vi "ArduPilot GCS.vi"() -> ()   [LabVIEW 8.6]
uses:
  user32.dll
  EventHandlerEnum.ctl
  Engines/SettingsEngine/SettingsEngineEnum.ctl
  EnumComm.ctl
  Engines/LogEngine/EnumLog.ctl
  Engines/SpeachEngine/EnumSpeak.ctl
panel:
  out "IMU":bool
  out "Climb Rate":dbl(knob) scale=-10.0..10.0 scale format="%#.2g"
  out "Mode":string
  out "WP":i32
  out "DistanceWP":i32 format="%.0f m"
  out "UAV Longitude":dbl format="%.6g°"
  out "UAV Latitude":dbl format="%.6g°"
  out "Throttle":i32(slide) scale=0.0..125.0
  out "Battery":dbl(slide) scale=0.0..10.0
  out "error outint comp manually":errorcluster
  out "error out clen-up":errorcluster
  out "Roll-old":i32
  out "Pitch-old":i32
  in  "WebBrowser 2":refnum<k7>(container)
  in  "Heading":string="0"
  in  "Range":string="1000"
  in  "Tilt":string="0"
  in  "Send":bool
  in  "write buffer":string
  in  "Baud Rate":string(combo)="9600"
  in  "COM Port":refnum<visa-resource-name>
  out "Comm Status":bool
  in  "EARTHLib.IApplicationGE":refnum<k7>
  in  "EARTHLib.IKHInterface":refnum<k7>
  out "GPS fix":bool
  out "error out":errorcluster
  out "StatusMsg":string
  out "Ground Speed Num":i32 format="%.0f m/s"
  out "Air Speed Num":i32 format="%.0f m/s"
  in  "Stop":bool
  out "Est Time Left":i32
  out "Amps":i32
  out "Watts":i32
  out "log data":string
  in  "Tab Control":T1(tab)
  out "GndSpeed":i32(knob) scale=0.0..50.0
  out "AS":i32
  out "GS":i32
  out "AirSpeed":i32(knob) caption="Air Speed" scale=0.0..50.0
  out "Roll Ind":cluster{i32, i32}(knob)={0, 180} scale=0.0..360.0
  out "Pitch-pic":picture
  out "Course   Bearing":cluster{i32, i32}(knob) scale=0.0..360.0 scale format="%.0f°"
  out "Altitude":cluster{i32, i32}(knob) scale=0.0..200.0
  out "BER":i32
  out "CRS":i32
  out "ALT":i32
  out "ALH":i32
  out "Roll":i32
  out "Pitch":i32
  in  "Zoom":u16(slide)=1000 scale=60000.0..1.0
  in  "Tilt":u8(slide) scale=0.0..90.0
  in  "Connect":bool
  in  "Baud Rate -M":string(combo)="9600"
  in  "COM Port -M":refnum<visa-resource-name>
  in  "kml write interval [s]":u32=1
  in  "Announcement interval [sec]":u32=30
  in  "Pan":i16(knob) scale=0.0..359.0
  out "IMU Performance data":string
  out "IMU health":i32
  out "Debug / Not Telemetry Data":string
  out "Raw Data":string
  # "NOT USED"
  # "%%%PWP:\t\t376322464,\t-1224913280,\t300,\nNWP:0,\t376321530,\t-1224913400,\t1200,***"
  # "meters"
  # "Climb Rate"
  # "lon 122\nlat 37"
  # "-122.491"
  # "37.6322"
  # "meters"
  # "ALH"
  # "m / s"
  # "meters"
  # "ALH"
  # "Gnd Speed"
  # "m/s"
  # "AP port - manuall connection"
  # "To manually connect to AP serial port\nselect desired 'COM port' and 'Boud Rate' values\nand press 'Connect'"
  # "Google Earth Controls"
  # "Audio"
  # "N"
  # "(How often to update kml (GE) display)"
  # "Received"
  # "Set"
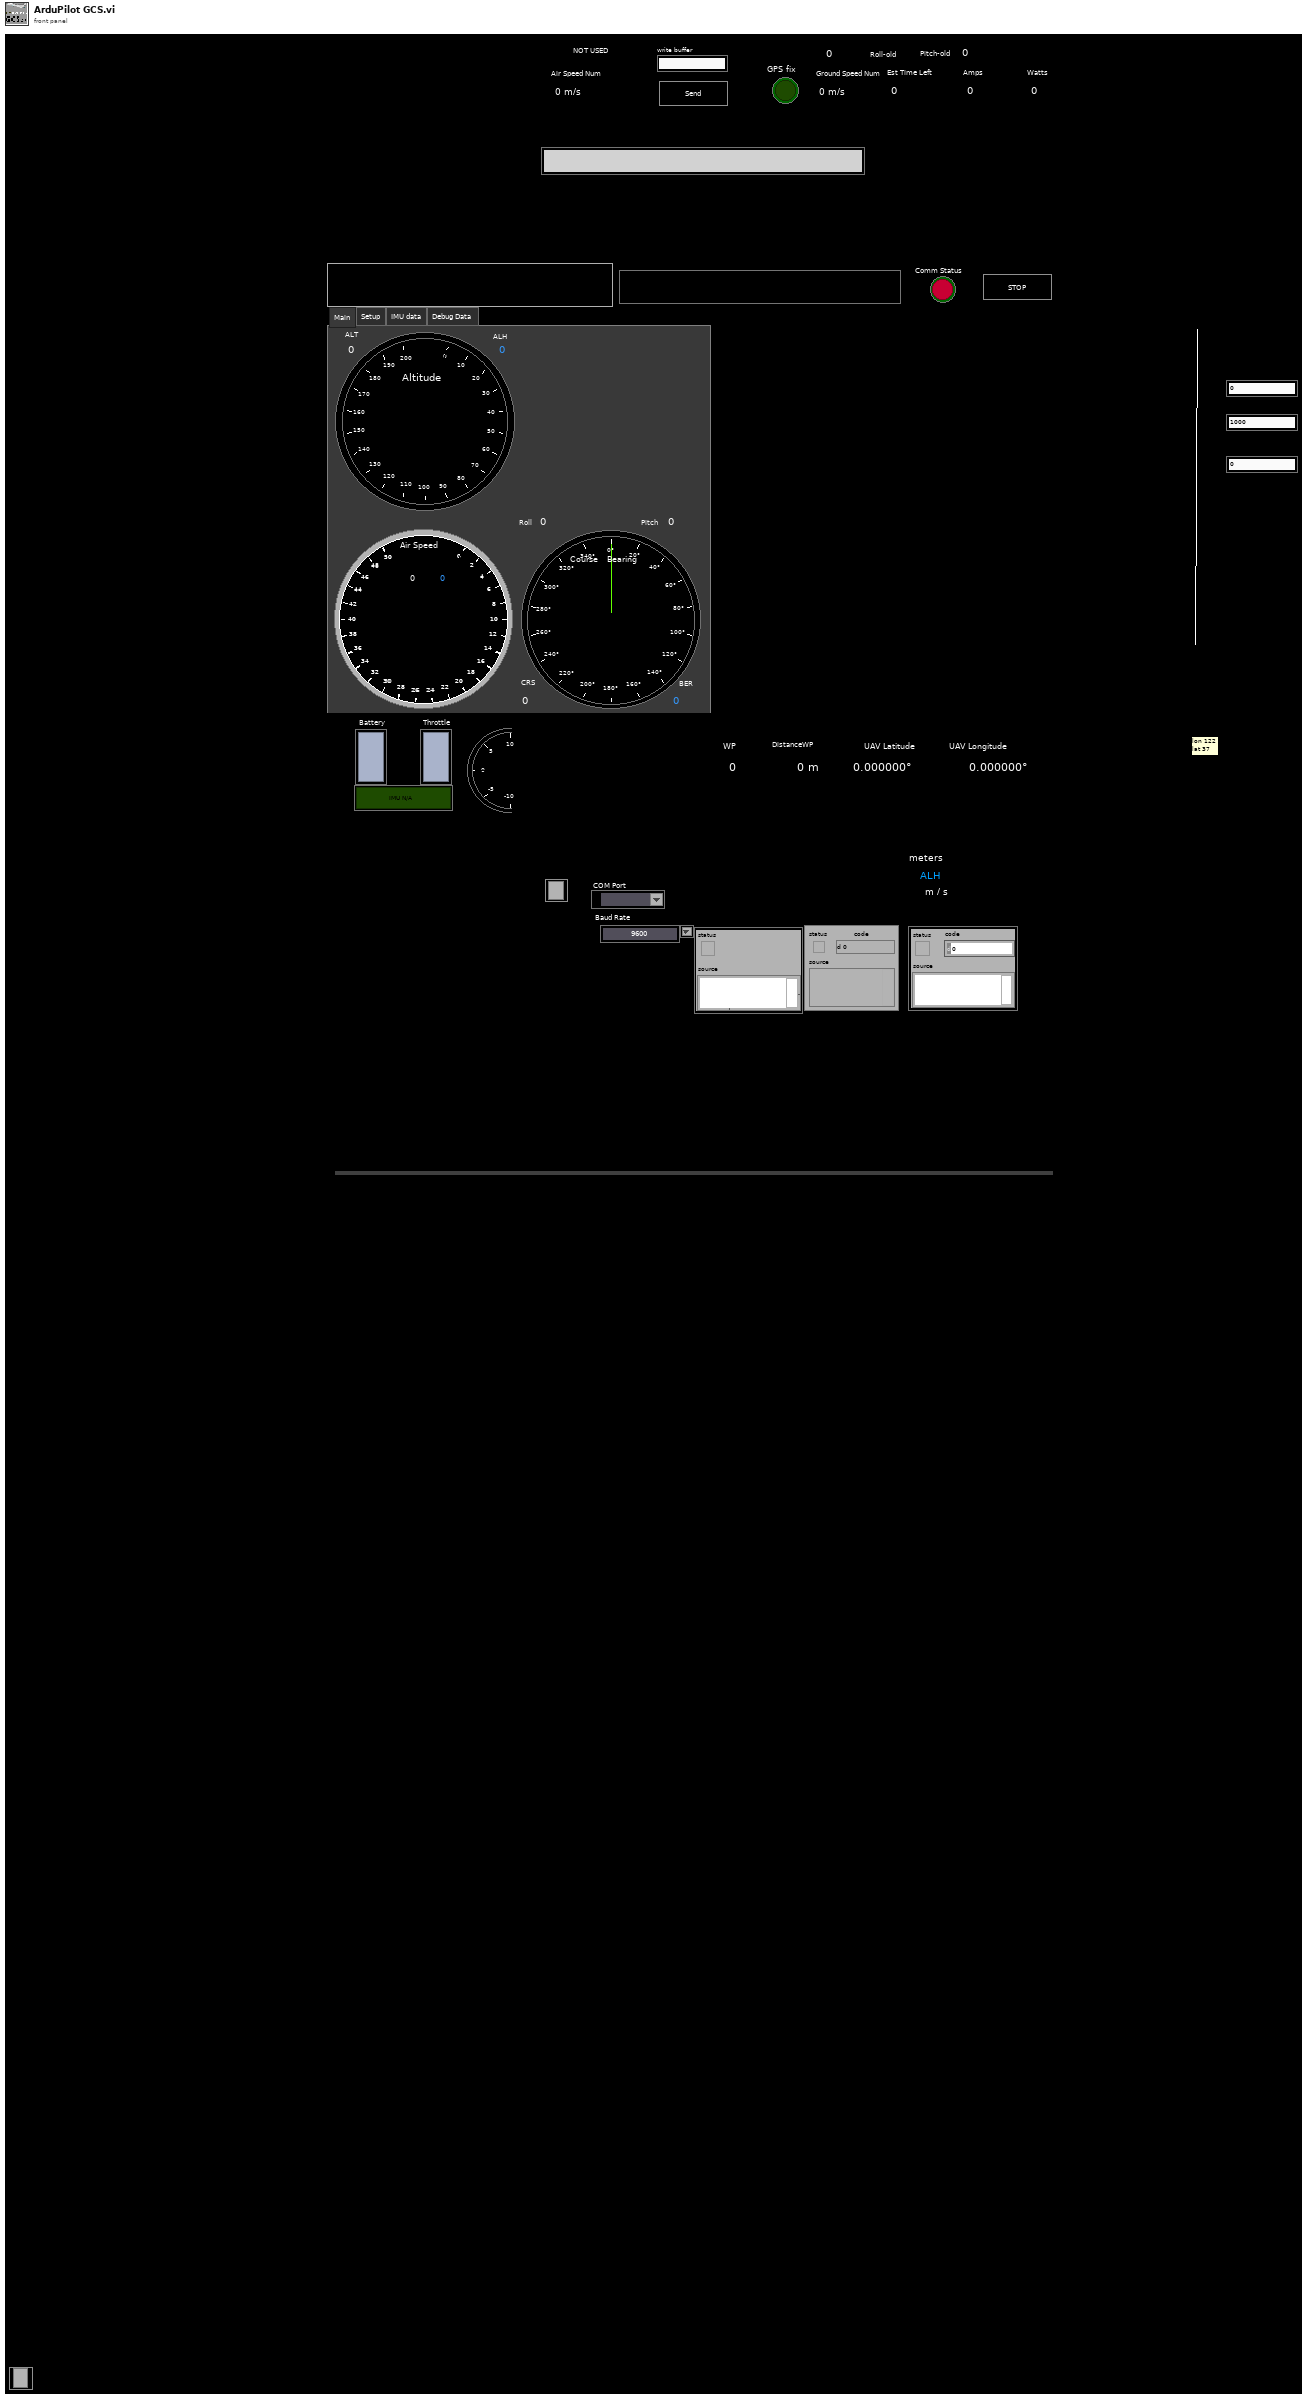
[diagram p1: front panel]
types:
  T1 = enum32{"Main", "Setup", "IMU data", "Debug Data"}
  T2 = typedef "EnumLog.ctl" = enum16{"Idle", "Log", "Init", "AddWP", "Stop", "CleanUp"}
  T3 = typedef "EnumComm.ctl" = enum16{"Read", "Idle", "Init", "InitComPort", "InitComPortManually", "Stop", "CleanUp", "Send"}
  T4 = typedef "EventHandlerEnum.ctl" = enum16{"Timeout", "Stop", "UpdateGEView", "UpdateCamData", "FPV_View_On", "UpdateIndicators"}
  T5 = typedef "EnumSpeak.ctl" = enum16{"Idle", "Init", "Speak", "Close"}
  T6 = cluster{"output number":i32, "output number":i32}
  T7 = typedef "SettingsEngineEnum.ctl" = enum16{"Init", "Load Settings from File", "Get Setting", "Set/Create Setting", "Save Settings to File"}
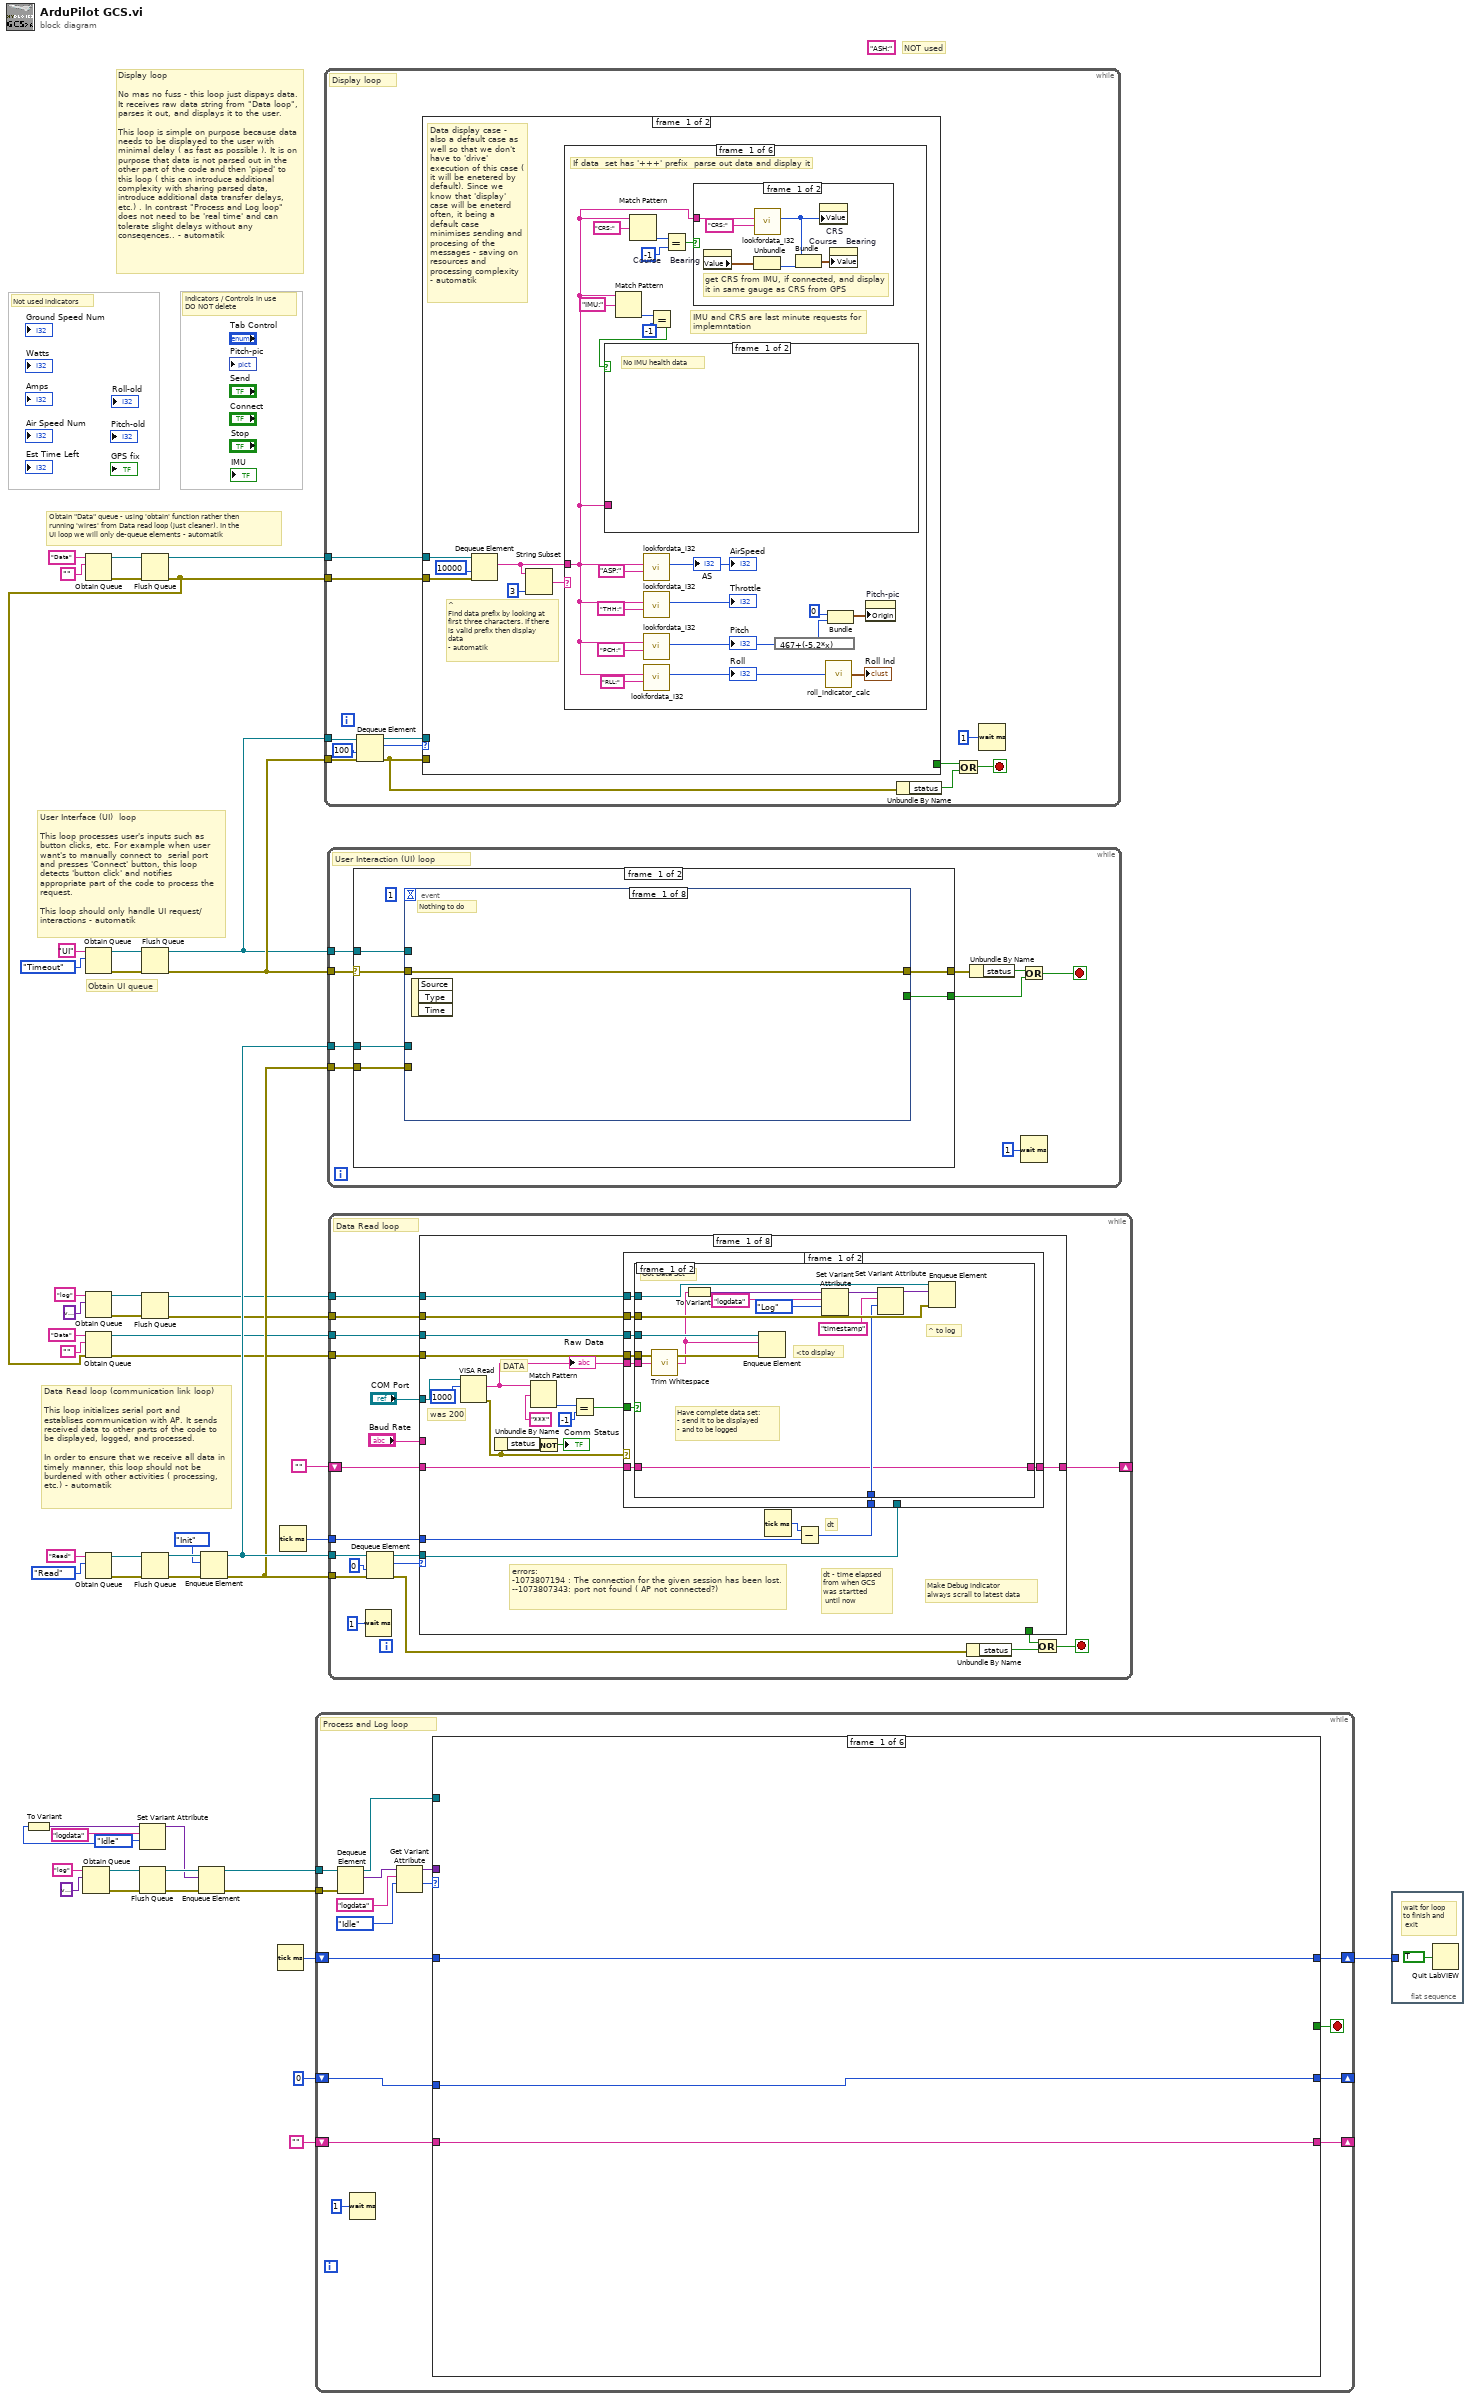
[diagram p0: block diagram]
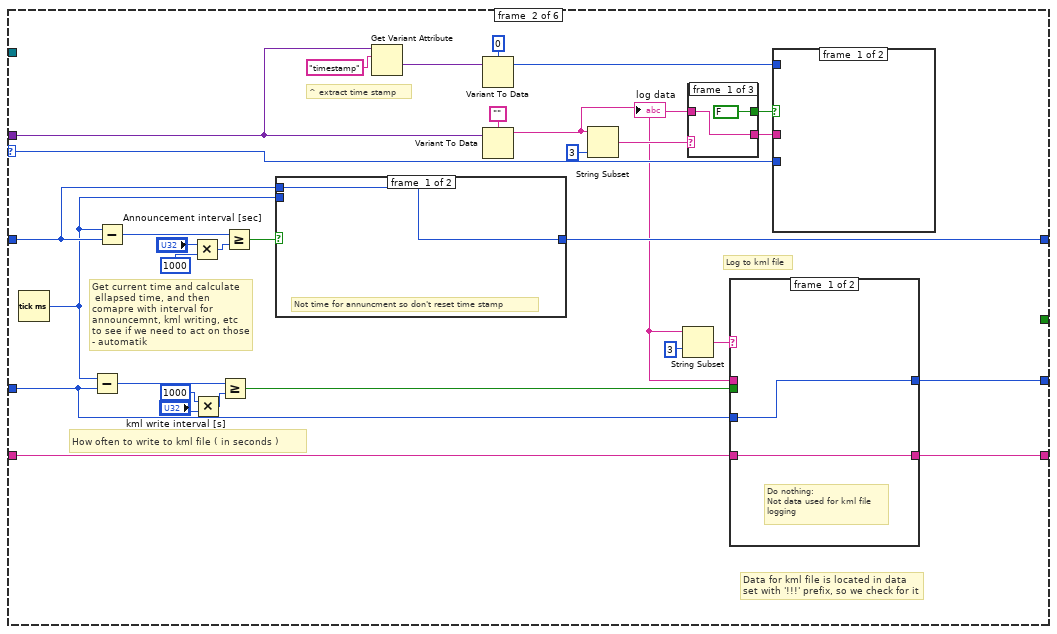
[diagram p2: hidden frame]
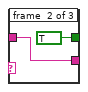
[diagram p3: hidden frame]
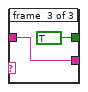
[diagram p4: hidden frame]
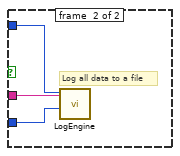
[diagram p5: hidden frame]
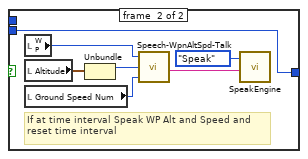
[diagram p6: hidden frame]
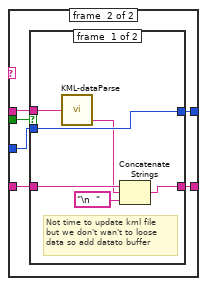
[diagram p7: hidden frame]
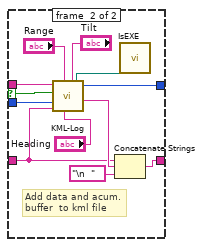
[diagram p8: hidden frame]
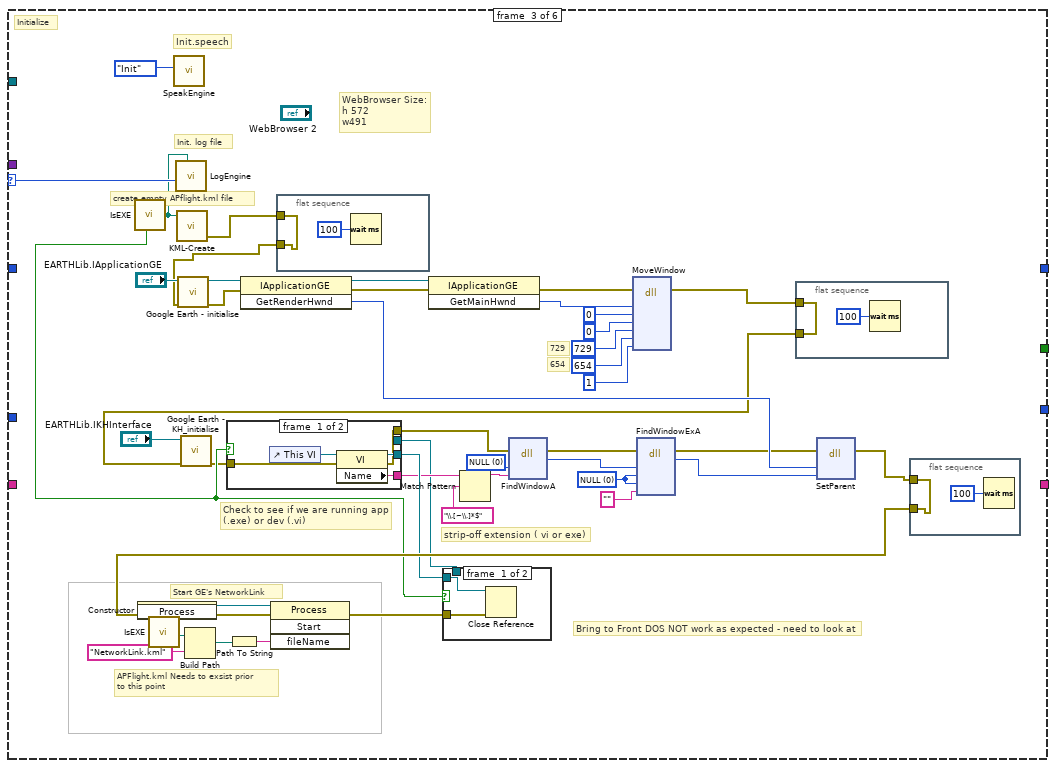
[diagram p9: hidden frame]
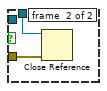
[diagram p10: hidden frame]
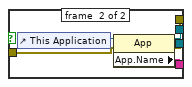
[diagram p11: hidden frame]
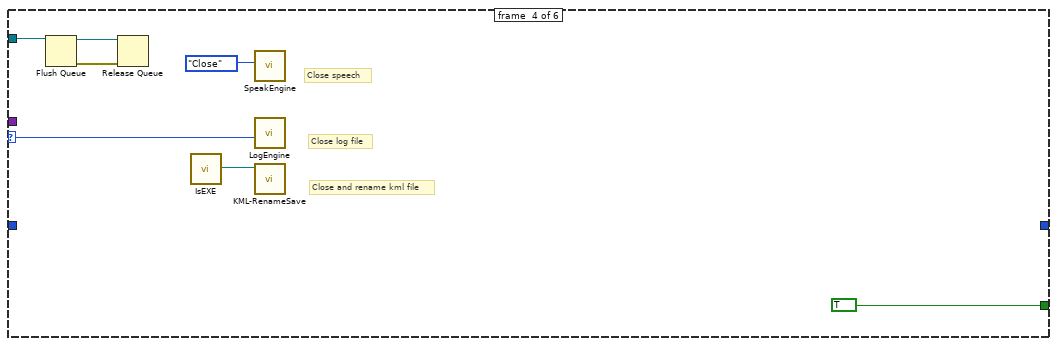
[diagram p12: hidden frame]
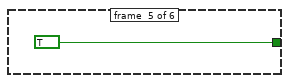
[diagram p13: hidden frame]
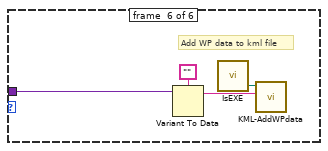
[diagram p14: hidden frame]
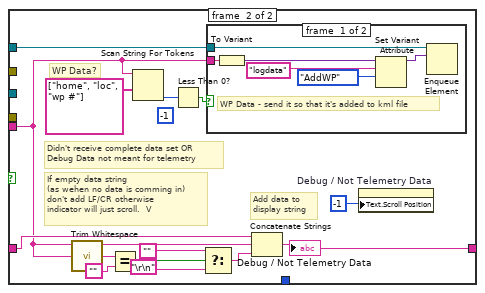
[diagram p15: hidden frame]
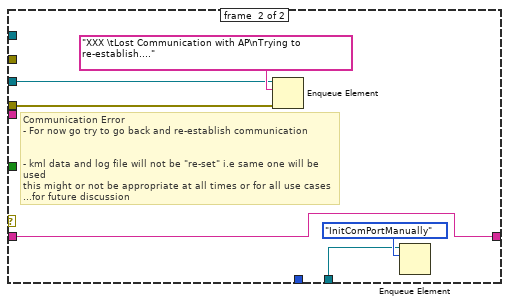
[diagram p17: hidden frame]
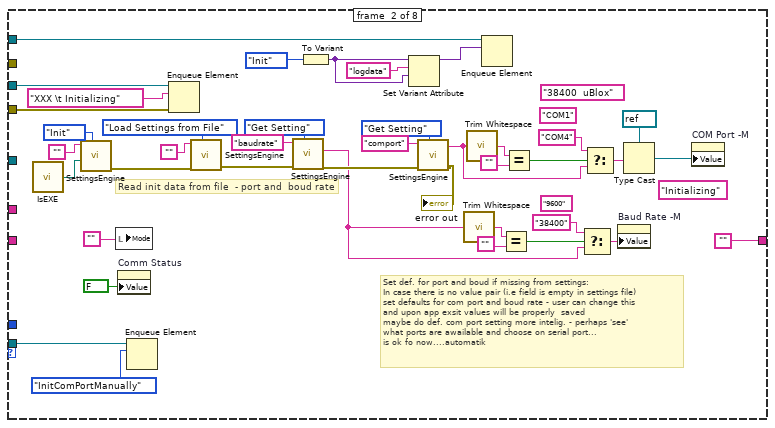
[diagram p18: hidden frame]
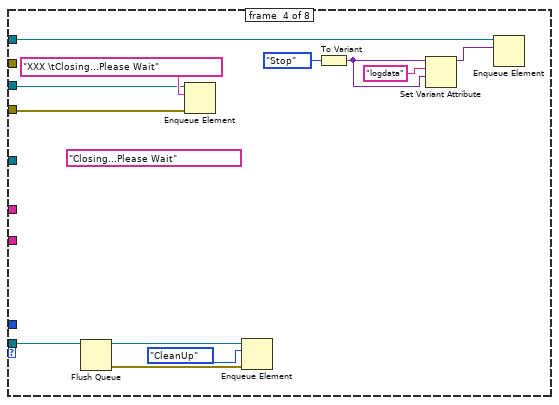
[diagram p20: hidden frame]
diagram:
  (unwired) "ASH:" ("regular expression")
  w11 = EnumLog."Idle" ("Log Enum")
  # "NOT used"
  # "Data Read loop (communication link loop)\n\nThis loop initializes serial port and establises communication with AP. It sends received data to other parts of the code to be displayed, logged, and processed.\n\nIn order to ensure that we receive all data in timely manner, this loop should not be burdened with other activities ( processing, etc.) - automatik"
  # "Obtain UI queue"
  # "User Interface (UI)  loop\n\nThis loop processes user's inputs such as button clicks, etc. For example when user want's to manually connect to  serial port and presses 'Connect' button, this loop detects 'button click' and notifies appropriate part of the code to process the request.\n\nThis loop should only handle UI request/ interactions - automatik"
  # "Obtain \"Data\" queue - using 'obtain' function rather then\nrunning 'wires' from Data read loop (just cleaner). In the\nUI loop we will only de-queue elements - automatik"
  # "Display loop\n\nNo mas no fuss - this loop just dispays data. It receives raw data string from \"Data loop\", parses it out, and displays it to the user. \n\nThis loop is simple on purpose because data needs to be displayed to the user with minimal delay ( as fast as possible ). It is on purpose that data is not parsed out in the other part of the code and then 'piped' to this loop ( this can introduce additional complexity with sharing parsed data, introduce additional data transfer delays, etc.) . In contrast \"Process and Log loop\"  does not need to be 'real time' and can tolerate slight delays without any conseqences.. - automatik"
  # "Indicators / Controls in use\nDO NOT delete"
  # "Not used indicators"
  n1 = To Variant(anything=w11) -> (Variant=w12:variant)
  n2 = Obtain Queue(name (unnamed)="log", element data type=variant ("variant")) -> (queue out=w18:refnum<queue>, error out=w6:errorcluster)  [unwired: 3 in, 1 out]
  n3 = Obtain Queue(name (unnamed)="Data", element data type="") -> (queue out=w28:refnum<queue>, error out=w26:errorcluster)  [unwired: 3 in, 1 out]
  n4 = Obtain Queue(name (unnamed)="UI", element data type=EventHandlerEnum."Timeout" ("Enum")) -> (queue out=w37:refnum<queue>, error out=w39:errorcluster)  [unwired: 3 in, 1 out]
  n5 = Obtain Queue(name (unnamed)="log", element data type=variant ("variant")) -> (queue out=w23:refnum<queue>, error out=w22:errorcluster)  [unwired: 3 in, 1 out]
  n6 = Obtain Queue(name (unnamed)="Read", element data type=EnumComm."Read" ("Comm Enum")) -> (queue out=w47:refnum<queue>, error out=w46:errorcluster)  [unwired: 3 in, 1 out]
  n7 = Set Variant Attribute(Variant=w12, name="logdata", value=w11) -> (Variant out=w10:variant)  [unwired: 1 in, 2 out]
  n8 = Flush Queue(queue=w18, error in (no error)=w6) -> (queue out=w15:refnum<queue>, error out=w4:errorcluster)  [unwired: 1 out]
  n9 = Flush Queue(queue=w28, error in (no error)=w26) -> (queue out=w27:refnum<queue>, error out=w25:errorcluster)  [unwired: 1 out]
  n10 = Obtain Queue(name (unnamed)="Data", element data type="", error in (no error)=w25) -> (queue out=w30:refnum<queue>, error out=w29:errorcluster)  [unwired: 2 in, 1 out]
  n11 = Flush Queue(queue=w37, error in (no error)=w39) -> (queue out=w36:refnum<queue>, error out=w38:errorcluster)  [unwired: 1 out]
  n12 = Flush Queue(queue=w23, error in (no error)=w22) -> (queue out=w21:refnum<queue>, error out=w20:errorcluster)  [unwired: 1 out]
  n13 = Flush Queue(queue=w47, error in (no error)=w46) -> (queue out=w45:refnum<queue>, error out=w44:errorcluster)  [unwired: 1 out]
  n14 = Enqueue Element(queue=w15, element=w10, error in (no error)=w4) -> (queue out=w14:refnum<queue>, error out=w3:errorcluster)  [unwired: 1 in, 1 out]
  n15 = Enqueue Element(queue=w45, element=EnumComm."Init" ("Comm Enum"), error in (no error)=w44) -> (queue out=w41:refnum<queue>, error out=w40:errorcluster)  [unwired: 1 in, 1 out]
  n16 = Tick Count (ms)() -> (millisecond timer value=w5:u32)
  n17 = Tick Count (ms)() -> (millisecond timer value=w9:u32)
  n18 = while {
    tunnel: w14 -> [w50]
    tunnel: w3 -> [w65]
    shift-right: [w58] -> _
    shift-left: "" -> [w57]
    shift-right: [w56] -> _
    shift-left: u32 0 ("millisecond timer value") -> [w55]
    shift-right: [w52] -> w1
    shift-left: w5 -> [w53]
    stop <- w60 stop-if-true
    # "Process and Log loop"
    n19 = Dequeue Element(queue=w50, error in (no error)=w65) -> (queue out=w51:refnum<queue>, element=w64:variant)  [unwired: 1 in, 2 out]
    n20 = Wait (ms)(milliseconds to wait=u32 1) -> ()  [unwired: 1 out]
    n21 = Get Variant Attribute(Variant=w64, name="logdata", default value (empty Variant)=EnumLog."Idle" ("Log Enum")) -> (duplicate Variant=w61:variant, value=w62:T2)  [unwired: 1 in, 2 out]
    n22 = case shown="\"Init\"" w62 {
      selector: w62 -> [_ w89 w183 w213 _ _]
      tunnel: w61 -> [_ w98 _ _ _ w218]
      tunnel: [_ _ _ TRUE ("x") TRUE ("x") _] -> w60
      tunnel: [w67 w92 _ _ _ _] -> w58
      tunnel: w57 -> [w67 w91 _ _ _ _]
      tunnel: [w68 w90 _ _ _ _] -> w56
      tunnel: w55 -> [w68 w88 _ _ _ _]
      tunnel: w53 -> [w66 w77 _ _ _ _]
      tunnel: [w66 w75 _ _ _ _] -> w52
      tunnel: w51 -> [_ _ _ w209 _ _]
      frame #0 {
      }
      frame #1 {
        # "Get current time and calculate\n ellapsed time, and then comapre with interval for announcemnt, kml writing, etc to see if we need to act on those - automatik"
        # "Data for kml file is located in data\nset with '!!!' prefix, so we check for it"
        # "^ extract time stamp"
        # "Log to kml file"
        # "How often to write to kml file ( in seconds )"
        n23 = Tick Count (ms)() -> (millisecond timer value=w76:u32)
        n24 = Subtract(x=w76, y=w88) -> (x-y=w93:u32)
        n25 = Subtract(x=w76, y=w77) -> (x-y=w79:u32)
        n26 = Multiply(x="Announcement interval [sec]", y=u32 1000) -> (x*y=w80:u32)
        n27 = Multiply(x=u32 1000, y="kml write interval [s]") -> (x*y=w84:u32)
        n28 = Greater Or Equal?(x=w93, y=w84) -> (x >= y?=w87:bool)
        n29 = Greater Or Equal?(x=w79, y=w80) -> (x >= y?=w78:bool)
        n30 = case shown="True" w78 {
          tunnel: w77 -> [w109 _]
          tunnel: w76 -> [_ w110]
          tunnel: [w109 w110] -> w75
          frame #0 {
            # "Not time for annuncment so don't reset time stamp"
          }
          frame #1 {
            # "If at time interval Speak WP Alt and Speed and reset time interval"
            n31 = local read "WP"() -> (w114:i32)
            n32 = local read "Altitude"() -> (w113:cluster{i32, i32})
            n33 = local read "Ground Speed Num"() -> (w116:i32)
            n34 = Unbundle(w113) -> (w115:i32)  [unwired: 1 out]
            n35 = call "Speech-WpnAltSpd-Talk.vi"("Ground Speed"=w116, "Numeric"=w115, "Current WP"=w114) -> ("Text"=w112:string)
            n36 = call "SpeakEngine.vi"("Text to speak"=w112, "EnumSpeak"=EnumSpeak."Speak") -> ()  [unwired: 9 in, 1 out]
          }
        }
        n37 = Get Variant Attribute(Variant=w98, name="timestamp") -> (value=w96:variant)  [unwired: 2 in, 3 out]
        n38 = Variant To Data(Variant=w96, type=u32 0 ("x-y 2")) -> (data=w94:u32)  [unwired: 1 in, 1 out]
        n39 = Variant To Data(Variant=w98, type="") -> (data=w70:string)  [unwired: 1 in, 1 out]
        "log data" <- w70
        n40 = String Subset(string=w70, length (rest)=3 ("length (rest)")) -> (substring=w71:string)  [unwired: 1 in]
        n41 = String Subset(string=w70, length (rest)=3 ("length (rest)")) -> (substring=w85:string)  [unwired: 1 in]
        n42 = case shown="\"+++\"" w71 {
          tunnel: [w100 w102 w104] -> w74
          tunnel: [FALSE TRUE TRUE] -> w73
          tunnel: w70 -> [w100 w102 w104]
          frame #0 {
          }
          frame #1 {
          }
          frame #2 {
          }
        }
        n43 = case shown="\"!!!\"" w85 {
          tunnel: [w117 w124] -> w92
          tunnel: w91 -> [w117 w123]
          tunnel: [w118 w122] -> w90
          tunnel: w88 -> [w118 w121]
          tunnel: w87 -> [_ w119]
          tunnel: w70 -> [_ w120]
          frame #0 {
            # "Do nothing:\nNot data used for kml file\nlogging"
          }
          frame #1 {
            n44 = case shown="True" w119 {
              selector: w119 -> [_ w134]
              tunnel: [w127 w141] -> w124
              tunnel: w123 -> [w128 w138]
              tunnel: [w129 w137] -> w122
              tunnel: w121 -> [w129 w136]
              tunnel: w120 -> [w126 w135]
              frame #0 {
                # "Not time to update kml file\nbut we don't wan't to loose\ndata so add datato buffer"
                n45 = call "KML-dataParse.vi"("data in"=w126) -> ("Cur loc (out)"=w125:string)  [unwired: 1 in, 1 out]
                n46 = Concatenate Strings(w128, w125, "\n  " ("string")) -> (w127:string)
              }
              frame #1 {
                # "Add data and acum. \nbuffer  to kml file"
                n47 = call "IsEXE.vi"() -> ("path to vi or exe install\\data\\ dir"=w140:path)  [unwired: 10 out]
                n48 = call "KML-Log.vi"("path to vi or exe (in)"=w140, "Tilt"="Tilt", "Heading"="Heading", "Range"="Range", "Coords (in)"=w138, "TimerIN (sh)"=w136, "WriteToFile?"=w134, "data in"=w135) -> ("Cur loc (out)"=w139:string, "Timer OUT (sh)"=w137:u32)  [unwired: 2 in]
                n49 = Concatenate Strings(w138, w139, "\n  " ("string")) -> (w141:string)
              }
            }
          }
        }
        n50 = case shown="True" w73 {
          tunnel: w94 -> [_ w108]
          tunnel: w89 -> [_ w107]
          tunnel: w74 -> [_ w106]
          frame #0 {
          }
          frame #1 {
            # "Log all data to a file"
            n51 = call "LogEngine.vi"("Log Enum"=w107, "LogDataIN"=w106, "cumul time"=w108) -> ()  [unwired: 9 in]
          }
        }
      }
      frame #2 {
        w171 = 0 items=["NULL"]
        w180 = 0 items=["NULL"]
        # "strip-off extension ( vi or exe)"
        # "Check to see if we are running app\n(.exe) or dev (.vi)"
        # "Bring to Front DOS NOT work as expected - need to look at"
        # "create empty APflight.kml file"
        # "WebBrowser Size:\nh 572\nw491"
        # "729"
        # "654"
        # "APFlight.kml Needs to exsist prior\nto this point"
        # "Start GE's NetworkLink"
        # "Init.speech"
        # "Init. log file"
        # "Initialize"
        n52 = call "IsEXE.vi"() -> ("path to vi or exe install\\data\\ dir"=w151:path, "is exe?"=w149:bool)  [unwired: 9 out]
        n53 = constructor class="Process"(error in=w152) -> (reference out=w160:refnum<k24>, error out=w159:errorcluster)  [unwired: 2 in, 1 out]
        n54 = call "IsEXE.vi"() -> ("path to vi or exe install\\data\\ dir"=w185:path)  [unwired: 10 out]
        n55 = call "SpeakEngine.vi"("EnumSpeak"=EnumSpeak."Init") -> ()  [unwired: 10 in, 1 out]
        n56 = call "LogEngine.vi"("dir path to file"=w151, "Log Enum"=w183) -> ()  [unwired: 10 in]
        n57 = call "KML-Create.vi"("path to vi or exe install\\data\\ dir"=w151) -> ("error out"=w155:errorcluster)  [unwired: 4 in]
        n58 = call "Google Earth - initialise.vi"("error in (no error)"=w154, "EARTHLib.IApplicationGE"="EARTHLib.IApplicationGE") -> ("error out"=w173:errorcluster, "Refnum Out"=w172:refnum<k7>)  [unwired: 8 out]
        n59 = call "Google Earth - KH_initialise.vi"("error in (no error)"=w156, "EARTHLib.IKHInterface"="EARTHLib.IKHInterface") -> ("error out"=w148:errorcluster)  [unwired: 9 out]
        n60 = Build Path(base path=w185, name or relative path="NetworkLink.kml") -> (appended path=w186:path)
        n61 = case shown="True" w149 {
          tunnel: [w196 w200] -> w145
          tunnel: [w195 _] -> w150
          tunnel: [_ w199] -> w143
          tunnel: w148 -> [w193 w198]
          tunnel: [w192 w197] -> w147
          frame #0 {
            n62 = control-ref of="This VI"() -> (w194:refnum<vi>)
            n63 = property class="VI"(reference=w194, error in=w193) -> (reference out=w195:refnum<vi>, error out=w192:errorcluster, "Name"=w196:string)
          }
          frame #1 {
            n64 = control-ref of="This Application"() -> (w201:refnum<vi>)
            n65 = property class="App"(reference=w201, error in=w198) -> (reference out=w199:refnum<vi>, error out=w197:errorcluster, "App.Name"=w200:string)
          }
        }
        n66 = Path To String(path=w186) -> (string=w182:string)
        n67 = invoke class="IApplicationGE" method="GetRenderHwnd"(reference=w172, error in=w173) -> (reference out=w169:refnum<k7>, error out=w168:errorcluster, "GetRenderHwnd"=w175:i32)  [unwired: 1 in]
        n68 = invoke class="Process" method="Start"(reference=w160, error in=w159, "fileName"=w182) -> (error out=w158:errorcluster)  [unwired: 1 in, 3 out]
        n69 = flat-sequence {
          tunnel: w155 -> [w204]
          tunnel: [w204] -> w154
          frame #0 {
            n70 = Wait (ms)(milliseconds to wait=u32 100) -> ()  [unwired: 1 out]
          }
        }
        n71 = invoke class="IApplicationGE" method="GetMainHwnd"(reference=w169, error in=w168) -> (error out=w161:errorcluster, "GetMainHwnd"=w163:i32)  [unwired: 1 in, 1 out]
        n72 = case shown="False" w149 {
          tunnel: w158 -> [w188 w190]
          tunnel: w150 -> [w189 _]
          tunnel: w143 -> [_ w191]
          frame #0 {
            n73 = Close Reference(reference=w189, error in (no error)=w188) -> ()  [unwired: 1 out]
          }
          frame #1 {
            n74 = Close Reference(reference=w191, error in (no error)=w190) -> ()  [unwired: 1 out]
          }
        }
        n75 = Match Pattern(string=w145, regular expression="\\.[~\\.]*$") -> (before substring=w144:string)  [unwired: 4 out]
        n76 = dll-call lib="user32.dll" fn="FindWindowA" label="FindWindow"(error in=w147, "lpszClassName"=w180, "lpszWindowName"=w144) -> (error out=w176:errorcluster, "hWnd"=w179:u32)  [unwired: 4 in, 1 out]
        n77 = dll-call lib="user32.dll" fn="MoveWindow"(error in=w161, "hWnd"=w163, "X"=u32 0, "Y"=0, "nWidth"=u32 729, "nHeight"=u32 654, "bRepaint"=u8 1) -> (error out=w157:errorcluster)  [unwired: 5 in, 5 out]
        n78 = dll-call lib="user32.dll" fn="FindWindowExA" label="Find Child"(error in=w176, "Parent HWND"=w179, "Child_After HWND"=w171, "lpszClassName"=w171, "lpszWindowName"="") -> (error out=w170:errorcluster, "hWnd"=w178:u32)  [unwired: 5 in, 2 out]
        n79 = flat-sequence {
          tunnel: w157 -> [w206]
          tunnel: [w206] -> w156
          frame #0 {
            n80 = Wait (ms)(milliseconds to wait=u32 100) -> ()  [unwired: 1 out]
          }
        }
        n81 = dll-call lib="user32.dll" fn="SetParent" label="Set Parent"(error in=w170, "hWndChild"=w175, "hWndNewParent"=w178) -> (error out=w153:errorcluster)  [unwired: 4 in, 2 out]
        n82 = flat-sequence {
          tunnel: w153 -> [w202]
          tunnel: [w202] -> w152
          frame #0 {
            n83 = Wait (ms)(milliseconds to wait=u32 100) -> ()  [unwired: 1 out]
          }
        }
      }
      frame #3 {
        # "Close speech"
        # "Close and rename kml file"
        # "Close log file"
        n84 = Flush Queue(queue=w209) -> (queue out=w211:refnum<queue>, error out=w210:errorcluster)  [unwired: 1 in, 1 out]
        n85 = Release Queue(queue=w211, error in (no error)=w210) -> ()  [unwired: 1 in, 3 out]
        n86 = call "IsEXE.vi"() -> ("path to vi or exe install\\data\\ dir"=w208:path)  [unwired: 10 out]
        n87 = call "SpeakEngine.vi"("EnumSpeak"=EnumSpeak."Close") -> ()  [unwired: 10 in, 1 out]
        n88 = call "LogEngine.vi"("Log Enum"=w213) -> ()  [unwired: 11 in]
        n89 = call "KML-RenameSave.vi"("path to vi or exe install\\data\\ dir"=w208) -> ()  [unwired: 11 in]
      }
      frame #4 {
      }
      frame #5 {
        # "Add WP data to kml file"
        n90 = Variant To Data(Variant=w218, type="") -> (data=w217:string)  [unwired: 1 in, 1 out]
        n91 = call "IsEXE.vi"() -> ("path to vi or exe install\\data\\ dir"=w216:path)  [unwired: 10 out]
        n92 = call "KML-AddWPdata.vi"("wp data in (raw)"=w217, "kml file dir path"=w216) -> ()  [unwired: 9 in, 1 out]
      }
    }
  }
  n93 = while {
    tunnel: w36 -> [w220]
    tunnel: w38 -> [w228]
    tunnel: w25 -> [w225]
    tunnel: w27 -> [w224]
    stop <- w229 stop-if-true
    # "Display loop"
    n94 = Dequeue Element(queue=w220, timeout in ms (-1)=100, error in (no error)=w228) -> (queue out=w221:refnum<queue>, element=w231:T4, error out=w223:errorcluster)  [unwired: 1 out]
    n95 = case shown="\"Timeout\", Default" w231 {
      tunnel: w223 -> [_ w327]
      tunnel: [_ TRUE ("x")] -> w230
      tunnel: w225 -> [w232 _]
      tunnel: w224 -> [w233 _]
      tunnel: w221 -> [_ w326]
      frame #0 {
        # "Data display case - also a default case as well so that we don't have to 'drive' execution of this case ( it will be enetered by default). Since we know that 'display' case will be eneterd often, it being a default case  minimises sending and procesing of the messages - saving on resources and processing complexity\n- automatik"
        # "^\nFind data prefix by looking at first three characters. If there is valid prefix then display data\n- automatik"
        n96 = Dequeue Element(queue=w233, timeout in ms (-1)=10000, error in (no error)=w232) -> (element=w236:string)  [unwired: 3 out]
        n97 = String Subset(string=w236, length (rest)=3 ("length (rest)")) -> (substring=w235:string)  [unwired: 1 in]
        n98 = case shown="\"+++\"" w235 {
          tunnel: w236 -> [w238 w285 w315 w317 w324 _]
          frame #0 {
            # "IMU and CRS are last minute requests for \nimplemntation"
            # "If data  set has '+++' prefix  parse out data and display it"
            n99 = Match Pattern(string=w238, regular expression="IMU:" ("Header")) -> (offset past match=w241:i32)  [unwired: 1 in, 3 out]
            n100 = Match Pattern(string=w238, regular expression="CRS:" ("Header")) -> (offset past match=w245:i32)  [unwired: 1 in, 3 out]
            n101 = call "lookfordata_i32.vi"("string (in)"=w238, "Header"="ASP:" ("regular expression")) -> ("output number"=→"AirSpeed" →"AS":i32)  [unwired: 4 in, 2 out]
            n102 = call "lookfordata_i32.vi"("string (in)"=w238, "Header"="THH:" ("regular expression")) -> ("output number"=→"Throttle":i32)  [unwired: 4 in, 2 out]
            n103 = call "lookfordata_i32.vi"("string (in)"=w238, "Header"="PCH:") -> ("output number"=w247:i32)  [unwired: 4 in, 2 out]
            "Pitch" <- w247
            n104 = call "lookfordata_i32.vi"("string (in)"=w238, "Header"="RLL:") -> ("output number"=w248:i32)  [unwired: 4 in, 2 out]
            "Roll" <- w248
            n105 = Equal?(x=w241, y=-1) -> (x = y?=w239:bool)
            n106 = case shown="False" w239 {
              tunnel: w238 -> [_ w259]
              frame #0 {
                # "No IMU health data"
              }
              frame #1 {
                # "Display IMU health"
                # "70% = 255*0.7"
                # "100% = 255*1"
                # "Color display for IMU health"
                n107 = call "lookfordata_i32.vi"("string (in)"=w259, "Header"="IMU:") -> ("output number"=w260:i32)  [unwired: 4 in, 2 out]
                "IMU health" <- w260
                n108 = In Range and Coerce(upper limit=u8 255, x=w260, lower limit=u8 178) -> (In Range?=w262:bool)  [unwired: 1 out]
                n109 = case shown="False" w262 {
                  tunnel: [w266 cluster{"Color Box":u32, "Color Box 2":u32}[] [{"Color Box"=1985280, "Color Box 2"=1985280}, {"Color Box"=40757, "Color Box 2"=40757}, {"Color Box"=1985280, "Color Box 2"=1985280}, {"Color Box"=6618880, "Color Box 2"=6618880}] ("Colors [4] 5")] -> w261
                  tunnel: w260 -> [w270 _]
                  frame #0 {
                    # "30%= 255 *0.3"
                    n110 = In Range and Coerce(upper limit=u8 178, x=w270, lower limit=u8 76) -> (In Range?=w267:bool)  [unwired: 1 out]
                    n111 = case shown="False" w267 {
                      tunnel: [cluster{"Color Box":u32, "Color Box 2":u32}[] [{"Color Box"=1985280, "Color Box 2"=1985280}, {"Color Box"=16711680, "Color Box 2"=16711680}, {"Color Box"=1985280, "Color Box 2"=1985280}, {"Color Box"=6618880, "Color Box 2"=6618880}] ("Colors [4] 5") cluster{"Color Box":u32, "Color Box 2":u32}[] [{"Color Box"=1985280, "Color Box 2"=1985280}, {"Color Box"=16774930, "Color Box 2"=16774930}, {"Color Box"=1985280, "Color Box 2"=1985280}, {"Color Box"=6618880, "Color Box 2"=6618880}] ("Colors [4] 5")] -> w266
                      frame #0 {
                        # "means data is\nfrom 0 -29 %"
                      }
                      frame #1 {
                      }
                    }
                  }
                  frame #1 {
                  }
                }
                n112 = property on="IMU" class="Bool (strict)"("Colors [4]"=w261) -> ()  [unwired: 2 in, 2 out]
              }
            }
            n113 = Equal?(x=w245, y=-1) -> (x = y?=w243:bool)
            n114 = case shown="True" w243 {
              tunnel: w238 -> [w278 _]
              frame #0 {
                # "get CRS from IMU, if connected, and display\nit in same gauge as CRS from GPS"
                n115 = property on="Course   Bearing" class="Knob (strict)"() -> ("Value"=w275:cluster{i32, i32})  [unwired: 2 in, 2 out]
                n116 = Unbundle(w275) -> (w274:i32)  [unwired: 1 out]
                n117 = call "lookfordata_i32.vi"("string (in)"=w278, "Header"="CRS:") -> ("output number"=w276:i32)  [unwired: 4 in, 2 out]
                n118 = Bundle("output number"=w276, w274) -> (w277:cluster{"output number":i32, i32})  [unwired: 1 in]
                n119 = property on="CRS" class="DigNum (strict)"("Value"=w276) -> ()  [unwired: 2 in, 2 out]
                n120 = property on="Course   Bearing" class="Knob (strict)"("Value"=w277) -> ()  [unwired: 2 in, 2 out]
              }
              frame #1 {
                # "No CRS from IMU"
              }
            }
            n121 = expression code="467+(-5.2*x)"(w247) -> (w251:i32)
            n122 = call "roll_indicator_calc.vi"("Roll (in)"=w248) -> ("Roll Indicator (out)"=→"Roll Ind":cluster{"Roll ctrl":i32, i32})  [unwired: 4 in]
            n123 = Bundle("Scrollbar 2"=0, "output number"=w251) -> (w252:cluster{"Scrollbar 2":i32, "output number":i32})  [unwired: 1 in]
            n124 = property on="Pitch-pic" class="Pict"("Origin"=w252) -> ()  [unwired: 2 in, 2 out]
          }
          frame #1 {
            # "lon 122\nlat 37"
            # "Extra sapce left here in\ncase we need to add things"
            # "If data  set has '!!!' prefix  parse out data and display it"
            # "was i16"
            n125 = call "lookfordata_i32.vi"("string (in)"=w285, "Header"="LAT:") -> ("output number"=w297:i32)  [unwired: 4 in, 2 out]
            n126 = call "lookfordata_i32.vi"("string (in)"=w285, "Header"="LON:") -> ("output number"=w293:i32)  [unwired: 4 in, 2 out]
            n127 = call "lookfordata_i32.vi"("string (in)"=w285, "Header"="ALT:" ("regular expression")) -> ("output number"=w281:i32)  [unwired: 4 in, 2 out]
            "ALT" <- w281
            n128 = call "lookfordata_i32.vi"("string (in)"=w285, "Header"="ALH:" ("regular expression")) -> ("output number"=w280:i32)  [unwired: 4 in, 2 out]
            "ALH" <- w280
            n129 = call "lookfordata_i32.vi"("string (in)"=w285, "Header"="CRS:") -> ("output number"=w284:i32)  [unwired: 4 in, 2 out]
            "CRS" <- w284
            n130 = call "lookfordata_i32.vi"("string (in)"=w285, "Header"="BER:") -> ("output number"=w283:i32)  [unwired: 4 in, 2 out]
            "BER" <- w283
            n131 = call "lookfordata_i32.vi"("string (in)"=w285, "Header"="SPD:") -> ("output number"=→"GndSpeed" →"GS":i32)  [unwired: 4 in, 2 out]
            n132 = call "lookfordata_i32.vi"("string (in)"=w285, "Header"="WPN:") -> ("output number"=→"WP":i32)  [unwired: 4 in, 2 out]
            n133 = call "lookfordata_i32.vi"("string (in)"=w285, "Header"="DST:") -> ("output number"=→"DistanceWP":i32)  [unwired: 4 in, 2 out]
            n134 = call "lookfordata_dbl.vi"("Header"="CRT:", "string (in)"=w285) -> ("output_dbl"=→"Climb Rate":dbl)  [unwired: 4 in, 1 out]
            n135 = call "lookfordata_dbl.vi"("Header"="BTV:", "string (in)"=w285) -> ("output_dbl"=→"Battery":dbl)  [unwired: 4 in, 1 out]
            n136 = To Double Precision Float(number=w297) -> (double precision float=w296:dbl)
            n137 = To Double Precision Float(number=w293) -> (double precision float=w294:dbl)
            n138 = Bundle("output number"=w281, "output number"=w280) -> (→"Altitude":T6)  [unwired: 1 out]
            n139 = Bundle("output number"=w284, "output number"=w283) -> (→"Course   Bearing":T6)  [unwired: 1 out]
            n140 = expression code="x/1000000"(w294) -> (→"UAV Longitude":dbl)
            n141 = expression code="x/1000000"(w296) -> (→"UAV Latitude":dbl)
          }
          frame #2 {
            # "If data  set has '###' prefix  parse out data and display it"
            n142 = Match Pattern(string=w315, regular expression="###") -> (after substring=w312:string)  [unwired: 1 in, 3 out]
            n143 = Match Pattern(string=w312, regular expression="***") -> (before substring=w310:string)  [unwired: 1 in, 3 out]
            n144 = Match Pattern(string=w310, regular expression="\t") -> (before substring=→"Mode":string)  [unwired: 1 in, 3 out]
          }
          frame #3 {
            # "If data  set has 'XXX' prefix  parse out data and display it"
            # "Look at better ways \n  for passing data to\nStatusMsg (I.e rewrite)"
            n145 = Match Pattern(string=w317, regular expression="XXX") -> (after substring=w320:string)  [unwired: 1 in, 3 out]
            n146 = Match Pattern(string=w320, regular expression="***") -> (before substring=w318:string)  [unwired: 1 in, 3 out]
            n147 = Match Pattern(string=w318, regular expression="\t") -> (after substring=→"StatusMsg":string)  [unwired: 1 in, 3 out]
          }
          frame #4 {
            # "If data  set has 'PPP' prefix  parse out data and display it"
            n148 = Match Pattern(string=w324, regular expression="PPP") -> (after substring=→"IMU Performance data":string)  [unwired: 1 in, 3 out]
          }
          frame #5 {
            # "Received data set:\n- does not have a valid prefix (bad data or incomplete data set)\n or \n- there is nothing to display\nor\n- data set has not been received yet so code has nothing to dispay"
          }
        }
      }
      frame #1 {
        # "User pressed STOP button:\n\n- Release UI queue\n- send \"True\" signal to exit the loop \n- clean-up things (if any)"
        n149 = Release Queue(queue=w326, error in (no error)=w327) -> ()  [unwired: 1 in, 3 out]
      }
    }
    n150 = Unbundle By Name(w223) -> ("status"=w227:bool)
    n151 = Or(x=w230, y=w227) -> (x .or. y?=w229:bool)
    n152 = Wait (ms)(milliseconds to wait=u32 1) -> ()  [unwired: 1 out]
  }
  n153 = while {
    tunnel: w36 -> [w337]
    tunnel: w38 -> [w332]
    tunnel: w41 -> [w331]
    tunnel: w40 -> [w330]
    stop <- w333 stop-if-true
    # "User Interaction (UI) loop"
    n154 = case shown="No Error" w332 {
      selector: w332 -> [w340 w397]
      tunnel: w337 -> [w343 _]
      tunnel: [w342 w397] -> w335
      tunnel: [w341 _] -> w334
      tunnel: w331 -> [w339 _]
      tunnel: w330 -> [w338 _]
      frame #0 {
        (unwired) 1
        n155 = event shown="[1] \"Stop\": Value Change" {
          selector: _ -> [_ _ _ _ _ _ _ _]
          dyn-events: _ -> [_ _ _ _ _ _ _ _]
          timeout: _ -> [_ _ _ _ _ _ _ _]
          tunnel: w343 -> [_ w348 w372 _ _ _ _ _]
          tunnel: w340 -> [w344 w350 w374 _ _ _ _ _]
          tunnel: [w344 w349 w373 _ _ _ _ _] -> w342
          tunnel: [_ w345 TRUE _ _ _ _ _] -> w341
          tunnel: w339 -> [_ w347 w371 w377 w385 _ _ _]
          tunnel: w338 -> [_ w346 w370 w376 w384 _ _ _]
          event #0 {
            # "Nothing to do"
            n156 = event-data() -> ()  [unwired: 1 in, 3 out]
          }
          event #1 {
            # "User pressed STOP button"
            # "User pressed STOP button\nso send message to all components\nthat we are stopping.\nWe don't want to relese queues here as there might be 'clean-up' activities in other loops.\n\nSend 'True' signal to exit UI loop ( we are done and are exiting app...)"
            n157 = event-data() -> ("NewVal"=w345:bool)  [unwired: 1 in, 5 out]
            n158 = case shown="True" w345 {
              tunnel: w350 -> [w351 w356]
              tunnel: [w351 w362] -> w349
              tunnel: w348 -> [_ w361]
              tunnel: w347 -> [_ w359]
              tunnel: w346 -> [_ w353]
              frame #0 {
              }
              frame #1 {
                # "Empty queues to ensure STOP case is acted upon and that there are no 'residual' msgs"
                n159 = Flush Queue(queue=w361, error in (no error)=w356) -> (queue out=w357:refnum<queue>, error out=w355:errorcluster)  [unwired: 1 out]
                n160 = Flush Queue(queue=w359, error in (no error)=w353) -> (queue out=w354:refnum<queue>, error out=w352:errorcluster)  [unwired: 1 out]
                n161 = Enqueue Element At Opposite End(queue=w357, element=EventHandlerEnum."Stop", error in (no error)=w355) -> (error out=w362:errorcluster)  [unwired: 1 in, 2 out]
                n162 = Enqueue Element At Opposite End(queue=w354, element=EnumComm."Stop" ("Comm Enum"), error in (no error)=w352) -> ()  [unwired: 1 in, 3 out]
              }
            }
          }
          event #2 {
            # "Empty queues to ensure this  case is acted upon and that there are no 'residual' msgs"
            # "User initiated App Close"
            # "User initated app close  so send message to all components\nthat we are stopping.\nWe don't want to relese queues here as there might be 'clean-up' activities in other loops.\n\nSend 'True' signal to exit UI loop ( we are done and are exiting app...)"
            n163 = event-data() -> ()  [unwired: 1 in, 2 out]
            n164 = Flush Queue(queue=w372, error in (no error)=w374) -> (queue out=w366:refnum<queue>, error out=w365:errorcluster)  [unwired: 1 out]
            n165 = Flush Queue(queue=w371, error in (no error)=w370) -> (queue out=w364:refnum<queue>, error out=w363:errorcluster)  [unwired: 1 out]
            n166 = Enqueue Element At Opposite End(queue=w366, element=EventHandlerEnum."Stop", error in (no error)=w365) -> (error out=w373:errorcluster)  [unwired: 1 in, 2 out]
            n167 = Enqueue Element At Opposite End(queue=w364, element=EnumComm."Stop" ("Comm Enum"), error in (no error)=w363) -> ()  [unwired: 1 in, 3 out]
          }
          event #3 {
            # "User changed COM port or baud rate and pressed 'Connect' button"
            # "If code is here it means that user changed value\nof comm port or baud rate, so we will flush all data \nfrom queue and go to reinitilize com port with new\nsettings"
            n168 = event-data() -> ("NewVal"=w375:bool)  [unwired: 1 in, 1 out]
            n169 = case shown="True" w375 {
              tunnel: w377 -> [_ w381]
              tunnel: w376 -> [_ w378]
              frame #0 {
                # "Get value of button press:\nIf 'False\" user released button ('up-click') - do nothing"
              }
              frame #1 {
                # "Get value of button press:\nIf 'True\" user pressed down on the button"
                n170 = Flush Queue(queue=w381, error in (no error)=w378) -> (queue out=w380:refnum<queue>, error out=w379:errorcluster)  [unwired: 1 out]
                n171 = Enqueue Element(queue=w380, element=EnumComm."InitComPortManually" ("Comm Enum"), error in (no error)=w379) -> ()  [unwired: 1 in, 3 out]
              }
            }
          }
          event #4 {
            # "Case NOT used \nright now"
            # "SENDING DATA TO AP COM PORT IS CURRENTLY NOT USED\nIt's here for custom debuging putposes"
            n172 = event-data() -> ("NewVal"=w383:bool)  [unwired: 1 in, 1 out]
            n173 = case shown="True" w383 {
              tunnel: w385 -> [_ w389]
              tunnel: w384 -> [_ w386]
              frame #0 {
                # "Get value of button press:\nIf 'False\" user released button ('up-click') - do nothing"
              }
              frame #1 {
                # "Send Data to AP"
                n174 = Flush Queue(queue=w389, error in (no error)=w386) -> (queue out=w388:refnum<queue>, error out=w387:errorcluster)  [unwired: 1 out]
                n175 = Enqueue Element(queue=w388, element=EnumComm."Send" ("Comm Enum"), error in (no error)=w387) -> ()  [unwired: 1 in, 3 out]
              }
            }
          }
          event #5 {
            n176 = event-data() -> ()  [unwired: 1 in, 1 out]
            n177 = Number To Decimal String(number="Zoom") -> (decimal integer string=w391:string)  [unwired: 1 in]
            n178 = property on="Range" class="Str"("Value"=w391) -> ()  [unwired: 2 in, 2 out]
          }
          event #6 {
            n179 = event-data() -> ()  [unwired: 1 in, 1 out]
            n180 = Number To Decimal String(number="Tilt") -> (decimal integer string=w393:string)  [unwired: 1 in]
            n181 = property on="Tilt" class="Str"("Value"=w393) -> ()  [unwired: 2 in, 2 out]
          }
          event #7 {
            n182 = event-data() -> ()  [unwired: 1 in, 1 out]
            n183 = Number To Decimal String(number="Pan") -> (decimal integer string=w395:string)  [unwired: 1 in]
            n184 = property on="Heading" class="Str"("Value"=w395) -> ()  [unwired: 2 in, 2 out]
          }
        }
      }
      frame #1 {
        # "Queue Error - will exit the loop"
      }
    }
    n185 = Unbundle By Name(w335) -> ("status"=w336:bool)
    n186 = Or(x=w336, y=w334) -> (x .or. y?=w333:bool)
    n187 = Wait (ms)(milliseconds to wait=u32 1) -> ()  [unwired: 1 out]
  }
  n188 = while {
    tunnel: w41 -> [w398]
    tunnel: w40 -> [w410]
    tunnel: w30 -> [w407]
    tunnel: w29 -> [w406]
    tunnel: w21 -> [w405]
    tunnel: w20 -> [w404]
    tunnel: w9 -> [w403]
    shift-right: [w400] -> _
    shift-left: "" -> [w399]
    stop <- w411 stop-if-true
    # "Data Read loop"
    n189 = Wait (ms)(milliseconds to wait=u32 1) -> ()  [unwired: 1 out]
    n190 = Dequeue Element(queue=w398, timeout in ms (-1)=0, error in (no error)=w410) -> (queue out=w401:refnum<queue>, element=w415:T3, error out=w408:errorcluster)  [unwired: 1 out]
    n191 = case shown="\"InitComPortManually\"" w415 {
      tunnel: w401 -> [w417 w524 _ w536 w559 w584 w612 _]
      tunnel: "COM Port" -> [w435 _ _ _ w544 _ _ w614]
      tunnel: [_ _ _ _ TRUE ("x") _ _ _] -> w413
      tunnel: w407 -> [w434 w491 _ w527 w554 w569 w610 _]
      tunnel: w406 -> [w433 w490 _ w526 w553 w571 w609 _]
      tunnel: w405 -> [w432 w493 _ w533 w542 _ _ _]
      tunnel: w404 -> [w431 _ _ _ _ _ _ _]
      tunnel: w403 -> [w430 _ _ _ _ _ _ _]
      tunnel: "Baud Rate" -> [_ _ _ _ w543 _ _ _]
      tunnel: [w423 "" _ _ _ _ _ _] -> w400
      tunnel: w399 -> [w422 _ _ _ _ _ _ _]
      frame #0 {
        # "errors:\n-1073807194 : The connection for the given session has been lost.\n--1073807343: port not found ( AP not connected?)"
        # "Make Debug indicator\nalways scrall to latest data"
        # "dt - time elapsed\nfrom when GCS\nwas startted\n until now"
        # "dt"
        # "DATA"
        # "was 200"
        n192 = VISA Read(VISA resource name=w435, byte count=u32 1000) -> (read buffer=w419:string, error out=w418:errorcluster)  [unwired: 1 in, 2 out]
        "Raw Data" <- w419
        n193 = Unbundle By Name(w418) -> ("status"=w421:bool)
        n194 = Match Pattern(string=w419, regular expression="***") -> (offset past match=w426:i32)  [unwired: 1 in, 3 out]
        n195 = Not(x=w421) -> (.not. x?=→"Comm Status":bool)
        n196 = Equal?(x=w426, y=-1) -> (x = y?=w424:bool)
        n197 = Tick Count (ms)() -> (millisecond timer value=w429:u32)
        n198 = Subtract(x=w429, y=w430) -> (x-y=w428:u32)
        n199 = case shown="No Error" w418 {
          tunnel: w434 -> [w445 w482]
          tunnel: w433 -> [w444 w481]
          tunnel: w432 -> [w443 _]
          tunnel: w431 -> [w442 _]
          tunnel: w428 -> [w441 _]
          tunnel: w424 -> [w440 _]
          tunnel: [w439 w480] -> w423
          tunnel: w422 -> [w438 w480]
          tunnel: w419 -> [w437 _]
          tunnel: w417 -> [_ w484]
          frame #0 {
            n200 = case shown="True" w440 {
              tunnel: w445 -> [w459 _]
              tunnel: w444 -> [w458 _]
              tunnel: w443 -> [w457 w464]
              tunnel: w442 -> [w456 _]
              tunnel: w441 -> [w449 _]
              tunnel: w437 -> [w448 w461]
              tunnel: [w446 w472] -> w439
              tunnel: w438 -> [w446 w473]
              frame #0 {
                # "Have complete data set:\n- send it to be displayed\n- and to be logged"
                # "Got Data Set"
                # "^ to log"
                # "<to display"
                n201 = call <vilib>:"Trim Whitespace.vi"("string"=w448) -> ("trimmed string"=w447:string)  [unwired: 1 in]
                n202 = To Variant(anything=w447) -> (Variant=w454:variant)
                n203 = Enqueue Element(queue=w459, element=w447, error in (no error)=w458) -> ()  [unwired: 1 in, 3 out]
                n204 = Set Variant Attribute(Variant=w454, name="logdata", value=EnumLog."Log" ("Log Enum")) -> (Variant out=w452:variant)  [unwired: 1 in, 2 out]
                n205 = Set Variant Attribute(Variant=w452, name="timestamp", value=w449) -> (Variant out=w450:variant)  [unwired: 1 in, 2 out]
                n206 = Enqueue Element(queue=w457, element=w450, error in (no error)=w456) -> ()  [unwired: 1 in, 3 out]
              }
              frame #1 {
                (unwired) -1 ("y")
                # "Didn't receive complete data set OR\nDebug Data not meant for telemetry"
                # "WP Data?"
                # "Add data to \ndisplay string"
                # "If empty data string \n(as wehen no data is comming in)\ndon't add LF/CR otherwise \nindicator will just scroll.  V"
                n207 = call <vilib>:"Trim Whitespace.vi"("string"=w461) -> ("trimmed string"=w471:string)  [unwired: 1 in]
                n208 = Equal?(x=w471, y="") -> (x = y?=w469:bool)
                n209 = Scan String For Tokens(7:string[] ["home", "loc", "wp #"] ("operators (none)"), 9:w461) -> (0:w460:i32)  [unwired: 4 in, 3 out]
                n210 = Less Than 0?(x=w460) -> (x < 0?=w463:bool)
                n211 = Select(t="", s=w469, f="\r\n") -> (s? t:f=w467:string)
                n212 = case shown="False" w463 {
                  tunnel: w464 -> [w476 _]
                  tunnel: w461 -> [w474 _]
                  frame #0 {
                    # "WP Data - send it so that it's added to kml file"
                    n213 = To Variant(anything=w474) -> (Variant=w478:variant)
                    n214 = Set Variant Attribute(Variant=w478, name="logdata", value=EnumLog."AddWP" ("Log Enum")) -> (Variant out=w475:variant)  [unwired: 1 in, 2 out]
                    n215 = Enqueue Element(queue=w476, element=w475) -> ()  [unwired: 2 in, 3 out]
                  }
                  frame #1 {
                  }
                }
                n216 = Concatenate Strings(w473, w461, w467) -> (w472:string)
                "Debug / Not Telemetry Data" <- w472
                n217 = property on="Debug / Not Telemetry Data" class="Str"("Text.Scroll Position"=-1) -> ()  [unwired: 2 in, 2 out]
              }
            }
          }
          frame #1 {
            # "Communication Error\n- For now go try to go back and re-establish communication\n\n\n- kml data and log file will not be \"re-set\" i.e same one will be used\nthis might or not be appropriate at all times or for all use cases\n...for future discussion"
            n218 = Enqueue Element(queue=w482, element="XXX \tLost Communication with AP\nTrying to re-establish...." ("Setting Name"), error in (no error)=w481) -> ()  [unwired: 1 in, 3 out]
            n219 = Enqueue Element(queue=w484, element=EnumComm."InitComPortManually" ("Comm Enum")) -> ()  [unwired: 2 in, 3 out]
          }
        }
      }
      frame #1 {
        (unwired) "Initializing" ("Setting Name")
        (unwired) "9600" ("t")
        (unwired) "COM1" ("t")
        (unwired) "38400  uBlox" ("Baud Rate 2")
        # "Set def. for port and boud if missing from settings:\nIn case there is no value pair (i.e field is empty in settings file)\nset defaults for com port and boud rate - user can change this\nand upon app exsit values will be properly  saved\nmaybe do def. com port setting more intelig. - perhaps 'see'\nwhat ports are awailable and choose on serial port...\nis ok fo now....automatik"
        # "Read init data from file  - port and  boud rate"
        n220 = call "IsEXE.vi"() -> ("path to vi or exe install\\data\\ dir"=w488:path)  [unwired: 10 out]
        n221 = call "SettingsEngine.vi"("Enum"=SettingsEngineEnum."Init", "Dir for Settings File"=w488, "Setting Name"="") -> ("error out"=w522:errorcluster)  [unwired: 7 in, 1 out]
        n222 = local write "Mode"("") -> ()
        n223 = property on="Comm Status" class="Bool (strict)"("Value"=FALSE ("Comm")) -> ()  [unwired: 2 in, 2 out]
        n224 = Enqueue Element(queue=w524, element=EnumComm."InitComPortManually" ("Comm Enum")) -> ()  [unwired: 2 in, 3 out]
        n225 = Enqueue Element(queue=w491, element="XXX \t Initializing" ("Setting Name"), error in (no error)=w490) -> ()  [unwired: 1 in, 3 out]
        n226 = call "SettingsEngine.vi"("Enum"=SettingsEngineEnum."Load Settings from File", "error in"=w522, "Setting Name"="") -> ("error out"=w521:errorcluster)  [unwired: 7 in, 1 out]
        n227 = call "SettingsEngine.vi"("Enum"=SettingsEngineEnum."Get Setting", "error in"=w521, "Setting Name"="baudrate") -> ("error out"=w520:errorcluster, "Setting Value"=w507:string)  [unwired: 7 in]
        n228 = To Variant(anything=EnumLog."Init" ("Log Enum")) -> (Variant=w495:variant)
        n229 = Set Variant Attribute(Variant=w495, name="logdata", value=w495) -> (Variant out=w494:variant)  [unwired: 1 in, 2 out]
        n230 = call "SettingsEngine.vi"("Enum"=SettingsEngineEnum."Get Setting", "error in"=w520, "Setting Name"="comport") -> ("error out"=→"error out":errorcluster, "Setting Value"=w502:string)  [unwired: 7 in]
        n231 = call <vilib>:"Trim Whitespace.vi"("string"=w507) -> ("trimmed string"=w510:string)  [unwired: 1 in]
        n232 = call <vilib>:"Trim Whitespace.vi"("string"=w502) -> ("trimmed string"=w505:string)  [unwired: 1 in]
        n233 = Enqueue Element(queue=w493, element=w494) -> ()  [unwired: 2 in, 3 out]
        n234 = Equal?(x=w510, y="") -> (x = y?=w508:bool)
        n235 = Equal?(x=w505, y="") -> (x = y?=w503:bool)
        n236 = Select(t="38400", s=w508, f=w507) -> (s? t:f=w506:string)
        n237 = Select(t="COM4", s=w503, f=w502) -> (s? t:f=w501:string)
        n238 = property on="Baud Rate -M" class="CmbBox"("Value"=w506) -> ()  [unwired: 2 in, 2 out]
        n239 = Type Cast(type=refnum<visa-resource-name> refnum ("VISA resource name"), x=w501) -> (*(type *) &x=w511:refnum<visa-resource-name>)
        n240 = property on="COM Port -M" class="VISAName"("Value"=w511) -> ()  [unwired: 2 in, 2 out]
      }
      frame #2 {
        # "NOT USED now\n( it was used for auto detection\nof AP com port...)"
      }
      frame #3 {
        (unwired) "Closing...Please Wait" ("Setting Name")
        n241 = Flush Queue(queue=w536) -> (queue out=w535:refnum<queue>, error out=w534:errorcluster)  [unwired: 1 in, 1 out]
        n242 = Enqueue Element(queue=w527, element="XXX \tClosing...Please Wait" ("Setting Name"), error in (no error)=w526) -> ()  [unwired: 1 in, 3 out]
        n243 = Enqueue Element(queue=w535, element=EnumComm."CleanUp" ("Comm Enum"), error in (no error)=w534) -> ()  [unwired: 1 in, 3 out]
        n244 = To Variant(anything=EnumLog."Stop" ("Log Enum")) -> (Variant=w529:variant)
        n245 = Set Variant Attribute(Variant=w529, name="logdata", value=w529) -> (Variant out=w530:variant)  [unwired: 1 in, 2 out]
        n246 = Enqueue Element(queue=w533, element=w530) -> ()  [unwired: 2 in, 3 out]
      }
      frame #4 {
        n247 = Flush Queue(queue=w554, error in (no error)=w553) -> (queue out=w556:refnum<queue>, error out=w555:errorcluster)  [unwired: 1 out]
        n248 = Flush Queue(queue=w559) -> (queue out=w558:refnum<queue>, error out=w557:errorcluster)  [unwired: 1 in, 1 out]
        n249 = Release Queue(queue=w556, error in (no error)=w555) -> (error out=w538:errorcluster)  [unwired: 1 in, 2 out]
        n250 = call "SettingsEngine.vi"("Enum"=SettingsEngineEnum."Set/Create Setting", "New Setting Value"=w544, "Setting Name"="comport") -> ("error out"=w550:errorcluster)  [unwired: 7 in, 1 out]
        n251 = Release Queue(queue=w558, error in (no error)=w557) -> (error out=w541:errorcluster)  [unwired: 1 in, 2 out]
        n252 = call "SettingsEngine.vi"("Enum"=SettingsEngineEnum."Set/Create Setting", "error in"=w550, "New Setting Value"=w543, "Setting Name"="baudrate") -> ("error out"=w545:errorcluster)  [unwired: 6 in, 1 out]
        n253 = VISA Flush I/O Buffer(VISA resource name=w544) -> (VISA resource name out=w562:refnum<visa-resource-name>, error out=w561:errorcluster)  [unwired: 1 in, 1 out]
        n254 = VISA Close(VISA resource name=w562, error in (no error)=w561) -> (error out=w540:errorcluster)
        "error out clen-up" <- w540
        n255 = call "SettingsEngine.vi"("Enum"=SettingsEngineEnum."Save Settings to File", "error in"=w545, "Setting Name"="a") -> ("error out"=w539:errorcluster)  [unwired: 7 in, 1 out]
        n256 = flat-sequence {
          tunnel: w542 -> [w563]
          tunnel: w541 -> [_]
          tunnel: w540 -> [_]
          tunnel: w539 -> [_]
          tunnel: w538 -> [_]
          frame #0 {
            # "Once everything finishes\nsend stop to log loop\n\n- could of used merge-errors\nbut didn't because I didn't\nwant to pass potential errors\nto logdata queue"
            n257 = To Variant(anything=EnumLog."Stop" ("Log Enum")) -> (Variant=w564:variant)
            n258 = Set Variant Attribute(Variant=w564, name="logdata", value=w564) -> (Variant out=w565:variant)  [unwired: 1 in, 2 out]
            n259 = Enqueue Element(queue=w563, element=w565) -> ()  [unwired: 2 in, 3 out]
          }
        }
      }
      frame #5 {
        w587 = u16 10 items=["1.0", "1.5", "2.0"] ("stop bits (10: 1 bit)")
        # "use \\r (0xD) as a terminator"
        n260 = Flush Queue(queue=w569, error in (no error)=w571) -> (queue out=w568:refnum<queue>, error out=w570:errorcluster)  [unwired: 1 out]
        n261 = VISA Open(duplicate session (F)=FALSE, VISA resource name="COM Port -M") -> (VISA resource name=w578:refnum<visa-resource-name>, error out=w577:errorcluster)  [unwired: 3 in]
        n262 = Decimal String To Number(string="Baud Rate -M") -> (number=w586:i32)  [unwired: 3 out]
        n263 = Flush Queue(queue=w584) -> (queue out=w582:refnum<queue>)  [unwired: 1 in, 2 out]
        n264 = Wait (ms)(milliseconds to wait=u32 10) -> ()  [unwired: 1 out]
        n265 = To Unsigned Long Integer(number=w586) -> (unsigned 32bit integer=w585:u32)
        n266 = call "VISA Configure Serial Port (Serial Instr).vi"("VISA resource name"=w578, "timeout (10sec)"=u32 2000, "termination char\n(0xA = '\\n' = LF)"=u8 13 ("termination char\n(0xA = '\\n' = LF)"), "Enable Termination\nChar (T)"=TRUE ("Enable Termination\nChar (T)"), "baud rate (9600)"=w585, "data bits (8)"=u16 8, "parity (0:none)"=enum16{"None", "Odd", "Even", "Mark", "Space"}."None", "error in (no error)"=w577, "stop bits (10: 1 bit)"=w587) -> ("VISA resource name out"=w579:refnum<visa-resource-name>, "error out"=w576:errorcluster)  [unwired: 5 in]
        n267 = case shown="No Error" w576 {
          selector: w576 -> [_ w601]
          tunnel: w582 -> [w598 w606]
          tunnel: w579 -> [w597 w605]
          tunnel: "Baud Rate -M" -> [w596 _]
          tunnel: [w595 w604] -> w574
          tunnel: w568 -> [w595 w604]
          tunnel: w570 -> [w594 w603]
          tunnel: [w594 w603] -> w575
          tunnel: ["XXX\tGCS Port Set" ("Setting Name") "XXX\tCould not set AP Com Port...\nis AP ON?)" ("Setting Name")] -> w573
          frame #0 {
            (unwired) "GCS Port Set" ("Setting Name")
            # "Communication established\nwith AP:\n-go to read data\n-init. proc.  and logging\n-display msg to user"
            # "Send msg to initialize data processing and logging\n(WAS here - moved)"
            n268 = local write "Baud Rate"(w596) -> ()
            n269 = local write "COM Port"(w597) -> ()
            n270 = Enqueue Element(queue=w598, element=EnumComm."Read" ("Comm Enum")) -> ()  [unwired: 2 in, 3 out]
          }
          frame #1 {
            # "Error - try connecting again"
            n271 = VISA Close(VISA resource name=w605, error in (no error)=w601) -> (error out=→"error outint comp manually":errorcluster)
            n272 = Enqueue Element(queue=w606, element=EnumComm."InitComPortManually" ("Comm Enum")) -> ()  [unwired: 2 in, 3 out]
          }
        }
        n273 = Enqueue Element(queue=w574, element=w573, error in (no error)=w575) -> ()  [unwired: 1 in, 3 out]
      }
      frame #6 {
        n274 = Enqueue Element(queue=w612, element=EnumComm."Idle" ("Comm Enum")) -> ()  [unwired: 2 in, 3 out]
        n275 = Enqueue Element(queue=w610, element="XXX\tCould not set AP Port...Try again ( is AP ON?)" ("Setting Name"), error in (no error)=w609) -> ()  [unwired: 1 in, 3 out]
      }
      frame #7 {
        (unwired) "SendingData" ("Setting Name")
        n276 = VISA Write(VISA resource name=w614, write buffer="write buffer") -> ()  [unwired: 1 in, 3 out]
      }
    }
    n277 = Unbundle By Name(w408) -> ("status"=w412:bool)
    n278 = Or(x=w413, y=w412) -> (x .or. y?=w411:bool)
  }
  n279 = flat-sequence {
    tunnel: w1 -> [_]
    frame #0 {
      # "wait for loop\nto finish and\n exit"
      n280 = Quit LabVIEW(quit? (T)=TRUE) -> ()
    }
  }
